vi "Read Max File Size.vi"(8 "error in (no error)":errorcluster, 11 "EHVIT Logger in":refnum<class "Logger.lvclass">) -> (0 "error out":errorcluster, 2 "Max File Size":i32, 3 "EHVIT Logger out":refnum<class "Logger.lvclass">)   [LabVIEW 2017, in "Logger.lvlib" / "Logger.lvclass"]
uses:
  Logger.lvclass
  Logger.lvclass/Logger.ctl
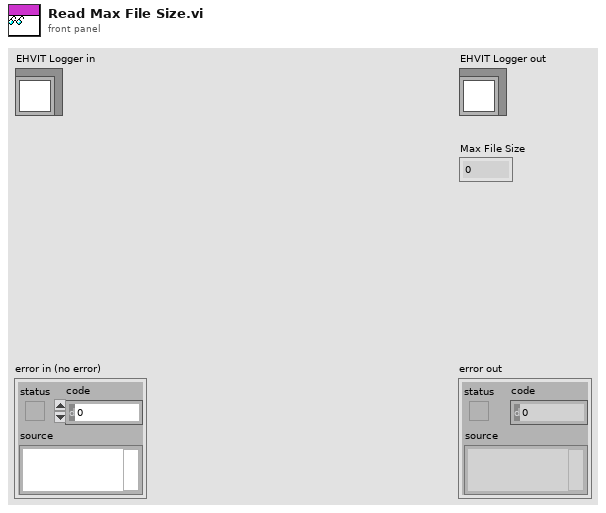
[diagram p1: front panel]
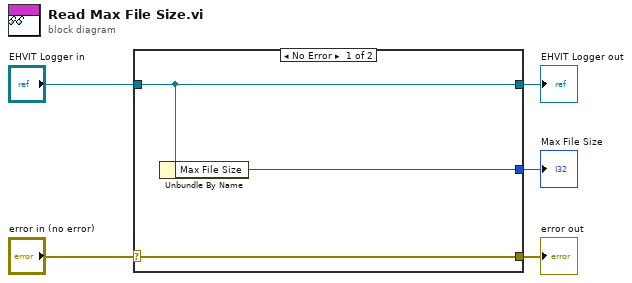
[diagram p0: block diagram]
diagram:
  n1 = case shown="No Error" "error in (no error)" {
    selector: "error in (no error)" -> [w8 w9]
    tunnel: [w8 w9] -> w4
    tunnel: [w7 w10] -> w2
    tunnel: "EHVIT Logger in" -> [w7 w10]
    tunnel: [w6 _] -> w1
    frame No Error {
      n2 = Unbundle By Name(w7) -> ("Max File Size"=w6:i32)
    }
    frame Error {
    }
  }
  "error out" <- w4
  "EHVIT Logger out" <- w2
  "Max File Size" <- w1
